vi "TC_alarm_Clusters_Sort_to_Numerics.vi"(11 "All_TC_ErrorStatus":T2) -> (3 "TC Alarms":T1)   [LabVIEW 2018]
uses:
  Controls/Clusts/All_TC_Error_Status.ctl
  Controls/Clusts/ErrorStatus.ctl
  TC_Data_Structure.ctl
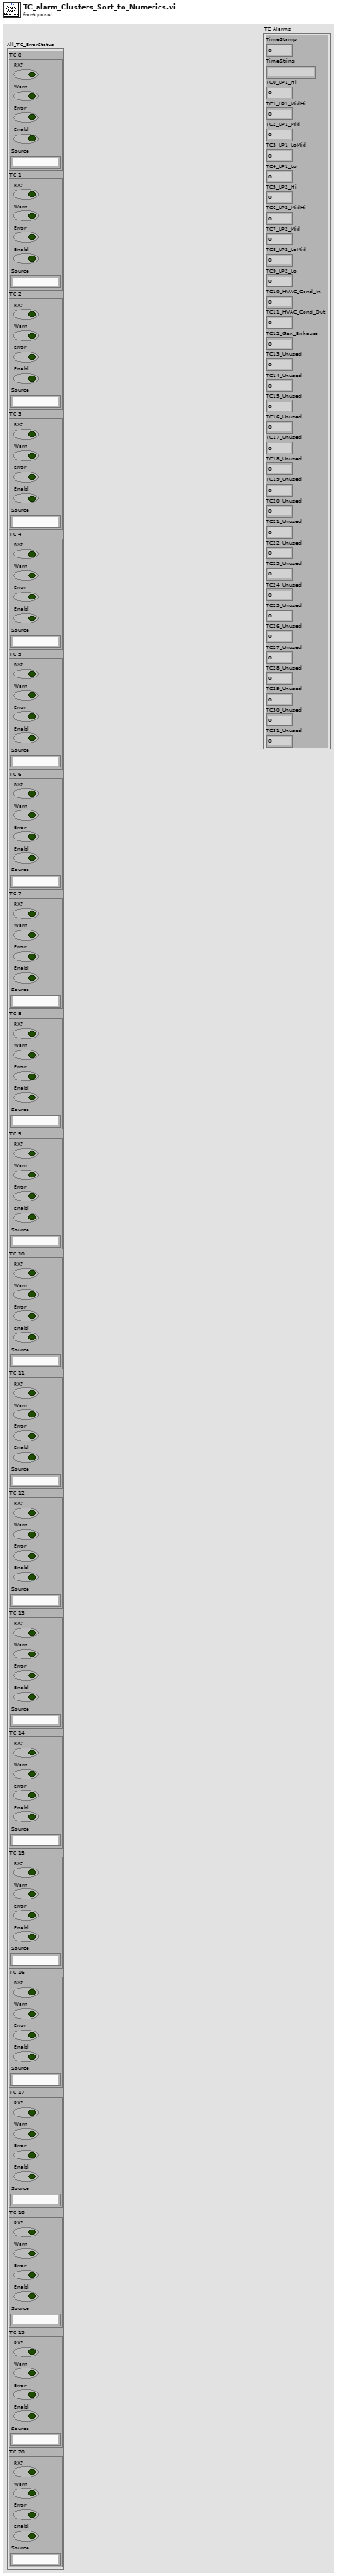
[diagram p1: front panel]
types:
  T1 = typedef "TC_Data_Structure.ctl" = cluster{"TimeStamp":dbl, "TimeString":string, "TC0_LP1_Hi":dbl, "TC1_LP1_MidHi":dbl, "TC2_LP1_Mid":dbl, "TC3_LP1_LoMid":dbl, "TC4_LP1_Lo":dbl, "TC5_LP2_Hi":dbl, "TC6_LP2_MidHi":dbl, "TC7_LP2_Mid":dbl, "TC8_LP2_LoMid":dbl, "TC9_LP2_Lo":dbl, "TC10_HVAC_Cond_In":dbl, "TC11_HVAC_Cond_Out":dbl, "TC12_Gen_Exhaust":dbl, "TC13_Unused":dbl, "TC14_Unused":dbl, "TC15_Unused":dbl, "TC16_Unused":dbl, "TC17_Unused":dbl, "TC18_Unused":dbl, "TC19_Unused":dbl, "TC20_Unused":dbl, "TC21_Unused":dbl, "TC22_Unused":dbl, "TC23_Unused":dbl, "TC24_Unused":dbl, "TC25_Unused":dbl, "TC26_Unused":dbl, "TC27_Unused":dbl, "TC28_Unused":dbl, "TC29_Unused":dbl, "TC30_Unused":dbl, "TC31_Unused":dbl}
  T2 = typedef "All_TC_Error_Status.ctl" = cluster{"TC 0":T3, "TC 1":T3, "TC 2":T3, "TC 3":T3, "TC 4":T3, "TC 5":T3, "TC 6":T3, "TC 7":T3, "TC 8":T3, "TC 9":T3, "TC 10":T3, "TC 11":T3, "TC 12":T3, "TC 13":T3, "TC 14":T3, "TC 15":T3, "TC 16":T3, "TC 17":T3, "TC 18":T3, "TC 19":T3, "TC 20":T3}
  T3 = typedef "ErrorStatus.ctl" = cluster{"RX?":bool, "Warn":bool, "Error":bool, "Enabl":bool, "Source":string}
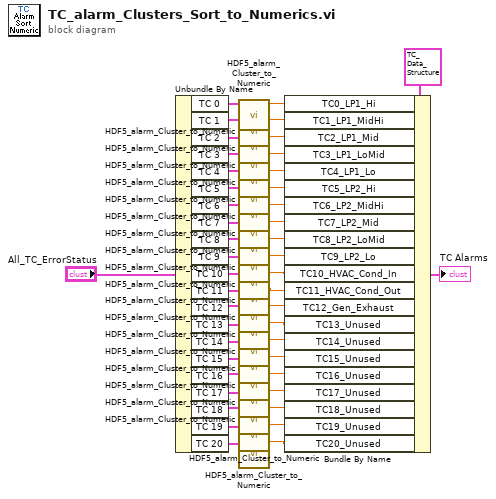
[diagram p0: block diagram]
diagram:
  n1 = Unbundle By Name("All_TC_ErrorStatus") -> ("TC 0"=w44:T3, "TC 1"=w22:T3, "TC 2"=w23:T3, "TC 3"=w24:T3, "TC 4"=w25:T3, "TC 5"=w26:T3, "TC 6"=w27:T3, "TC 7"=w28:T3, "TC 8"=w29:T3, "TC 9"=w30:T3, "TC 10"=w31:T3, "TC 11"=w32:T3, "TC 12"=w33:T3, "TC 13"=w34:T3, "TC 14"=w35:T3, "TC 15"=w36:T3, "TC 16"=w37:T3, "TC 17"=w38:T3, "TC 18"=w39:T3, "TC 19"=w40:T3, "TC 20"=w42:T3)
  n2 = call "HDF5_alarm_Cluster_to_Numeric.vi"("TC 0"=w44) -> ("f"=w45:dbl)  [unwired: 10 in]
  n3 = call "HDF5_alarm_Cluster_to_Numeric.vi"("TC 0"=w22) -> ("f"=w21:dbl)  [unwired: 10 in]
  n4 = call "HDF5_alarm_Cluster_to_Numeric.vi"("TC 0"=w23) -> ("f"=w20:dbl)  [unwired: 10 in]
  n5 = call "HDF5_alarm_Cluster_to_Numeric.vi"("TC 0"=w24) -> ("f"=w19:dbl)  [unwired: 10 in]
  n6 = call "HDF5_alarm_Cluster_to_Numeric.vi"("TC 0"=w25) -> ("f"=w18:dbl)  [unwired: 10 in]
  n7 = call "HDF5_alarm_Cluster_to_Numeric.vi"("TC 0"=w26) -> ("f"=w17:dbl)  [unwired: 10 in]
  n8 = call "HDF5_alarm_Cluster_to_Numeric.vi"("TC 0"=w27) -> ("f"=w16:dbl)  [unwired: 10 in]
  n9 = call "HDF5_alarm_Cluster_to_Numeric.vi"("TC 0"=w28) -> ("f"=w15:dbl)  [unwired: 10 in]
  n10 = call "HDF5_alarm_Cluster_to_Numeric.vi"("TC 0"=w29) -> ("f"=w14:dbl)  [unwired: 10 in]
  n11 = call "HDF5_alarm_Cluster_to_Numeric.vi"("TC 0"=w30) -> ("f"=w13:dbl)  [unwired: 10 in]
  n12 = call "HDF5_alarm_Cluster_to_Numeric.vi"("TC 0"=w31) -> ("f"=w12:dbl)  [unwired: 10 in]
  n13 = call "HDF5_alarm_Cluster_to_Numeric.vi"("TC 0"=w32) -> ("f"=w11:dbl)  [unwired: 10 in]
  n14 = call "HDF5_alarm_Cluster_to_Numeric.vi"("TC 0"=w33) -> ("f"=w10:dbl)  [unwired: 10 in]
  n15 = call "HDF5_alarm_Cluster_to_Numeric.vi"("TC 0"=w34) -> ("f"=w9:dbl)  [unwired: 10 in]
  n16 = call "HDF5_alarm_Cluster_to_Numeric.vi"("TC 0"=w35) -> ("f"=w8:dbl)  [unwired: 10 in]
  n17 = call "HDF5_alarm_Cluster_to_Numeric.vi"("TC 0"=w36) -> ("f"=w7:dbl)  [unwired: 10 in]
  n18 = call "HDF5_alarm_Cluster_to_Numeric.vi"("TC 0"=w37) -> ("f"=w6:dbl)  [unwired: 10 in]
  n19 = call "HDF5_alarm_Cluster_to_Numeric.vi"("TC 0"=w38) -> ("f"=w5:dbl)  [unwired: 10 in]
  n20 = call "HDF5_alarm_Cluster_to_Numeric.vi"("TC 0"=w39) -> ("f"=w4:dbl)  [unwired: 10 in]
  n21 = call "HDF5_alarm_Cluster_to_Numeric.vi"("TC 0"=w40) -> ("f"=w3:dbl)  [unwired: 10 in]
  n22 = call "HDF5_alarm_Cluster_to_Numeric.vi"("TC 0"=w42) -> ("f"=w41:dbl)  [unwired: 10 in]
  n23 = Bundle By Name(cluster=T1 {"TimeStamp"=0.0, "TimeString"="", "TC0_LP1_Hi"=0.0, "TC1_LP1_MidHi"=0.0, "TC2_LP1_Mid"=0.0, "TC3_LP1_LoMid"=0.0, "TC4_LP1_Lo"=0.0, "TC5_LP2_Hi"=0.0, "TC6_LP2_MidHi"=0.0, "TC7_LP2_Mid"=0.0, "TC8_LP2_LoMid"=0.0, "TC9_LP2_Lo"=0.0, "TC10_HVAC_Cond_In"=0.0, "TC11_HVAC_Cond_Out"=0.0, "TC12_Gen_Exhaust"=0.0, "TC13_Unused"=0.0, "TC14_Unused"=0.0, "TC15_Unused"=0.0, "TC16_Unused"=0.0, "TC17_Unused"=0.0, "TC18_Unused"=0.0, "TC19_Unused"=0.0, "TC20_Unused"=0.0, "TC21_Unused"=0.0, "TC22_Unused"=0.0, "TC23_Unused"=0.0, "TC24_Unused"=0.0, "TC25_Unused"=0.0, "TC26_Unused"=0.0, "TC27_Unused"=0.0, "TC28_Unused"=0.0, "TC29_Unused"=0.0, "TC30_Unused"=0.0, "TC31_Unused"=0.0} ("TCData"), "TC0_LP1_Hi"=w45, "TC1_LP1_MidHi"=w21, "TC2_LP1_Mid"=w20, "TC3_LP1_LoMid"=w19, "TC4_LP1_Lo"=w18, "TC5_LP2_Hi"=w17, "TC6_LP2_MidHi"=w16, "TC7_LP2_Mid"=w15, "TC8_LP2_LoMid"=w14, "TC9_LP2_Lo"=w13, "TC10_HVAC_Cond_In"=w12, "TC11_HVAC_Cond_Out"=w11, "TC12_Gen_Exhaust"=w10, "TC13_Unused"=w9, "TC14_Unused"=w8, "TC15_Unused"=w7, "TC16_Unused"=w6, "TC17_Unused"=w5, "TC18_Unused"=w4, "TC19_Unused"=w3, "TC20_Unused"=w41) -> (→"TC Alarms":T1)
